vi "Falling Edge Detector.vi"(1 "Input":bool) -> (0 "Falling edge?":bool)   [LabVIEW 2015]
doc: "Emits True when input changes from True -> False"
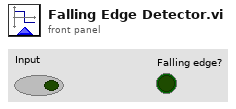
[diagram p1: front panel]
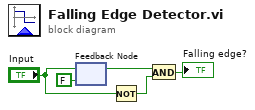
[diagram p0: block diagram]
diagram:
  n1 = feedback-in #1("Input") -> ()
  n2 = feedback #1(FALSE ("Input")) -> (w1:bool)
  n3 = Not(x="Input") -> (.not. x?=w3:bool)
  n4 = And(x=w1, y=w3) -> (x .and. y?=→"Falling edge?":bool)
